vi "z_N[Psi_tau,tau_0,T,W,t_0]_Analytical.vi"(4 "Use z[0]":bool, 5 "tau_0":ext, 6 "t0":ext, 7 "Harmonic f":ext, 8 "N":i32, 9 "W":ext, 10 "T":ext, 11 "tau":ext) -> (3 "z_n,N,W(tau,tau_0)":cxt)   [LabVIEW 2019]
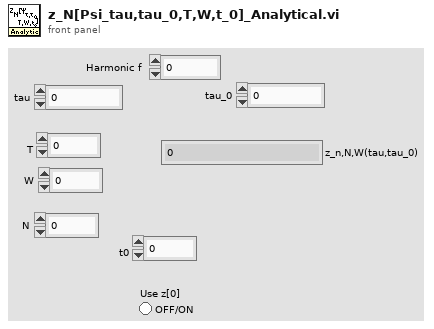
[diagram p1: front panel]
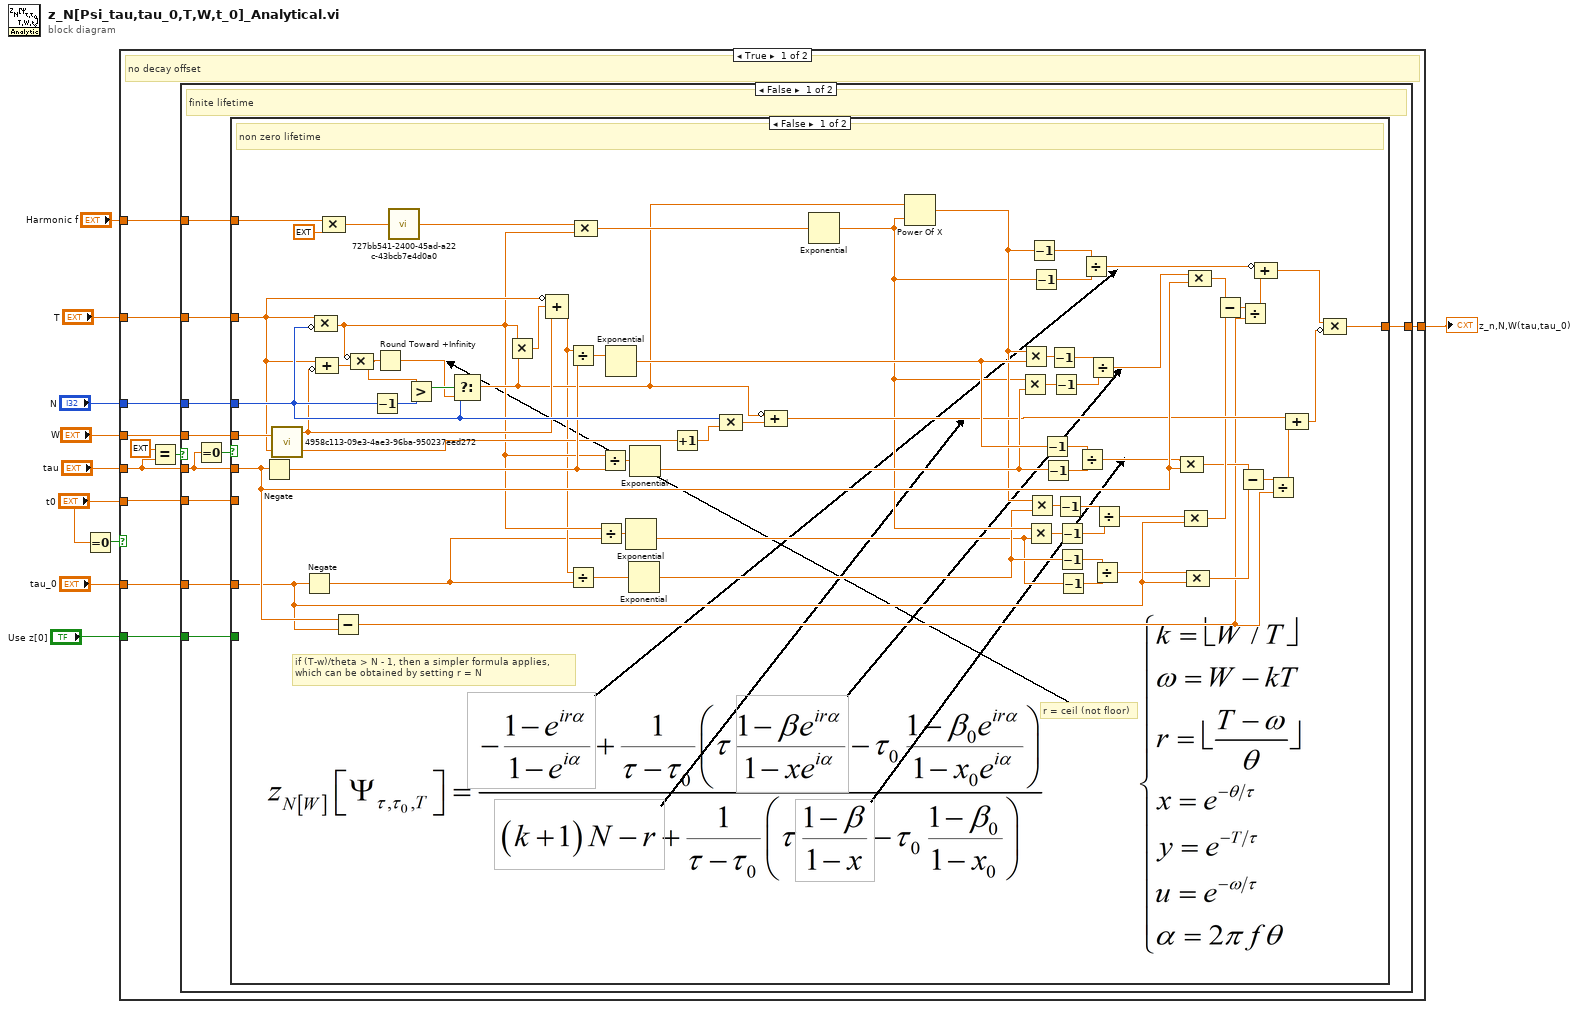
[diagram p0: block diagram]
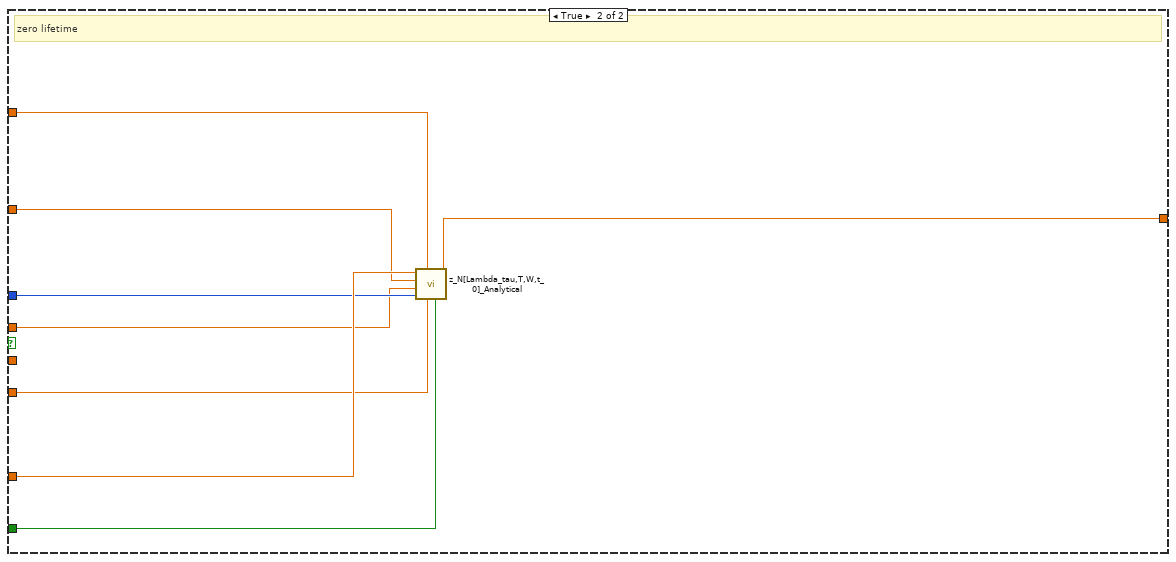
[diagram p2: hidden frame]
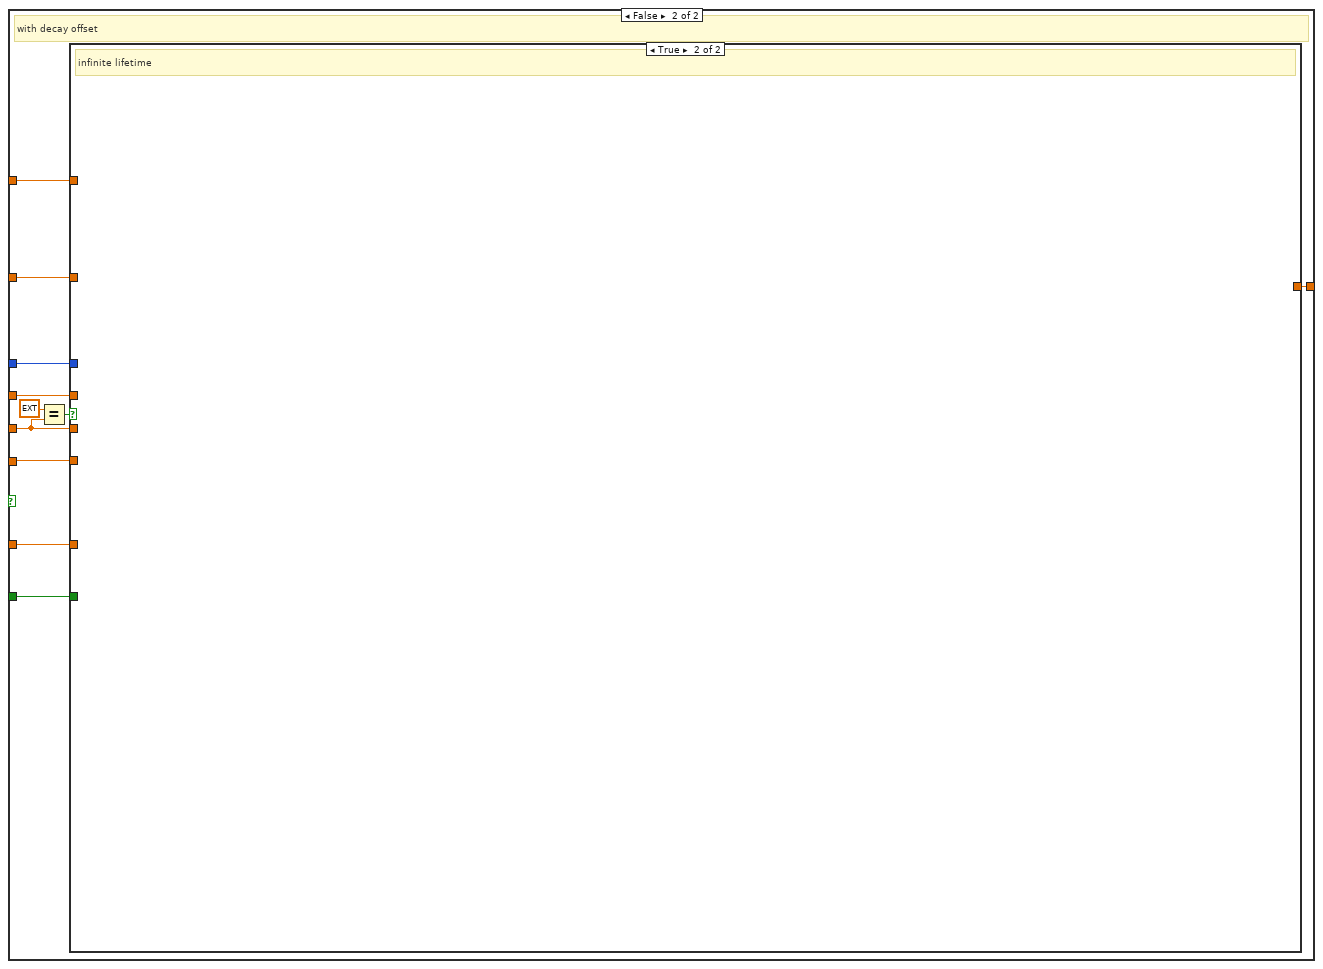
[diagram p4: hidden frame]
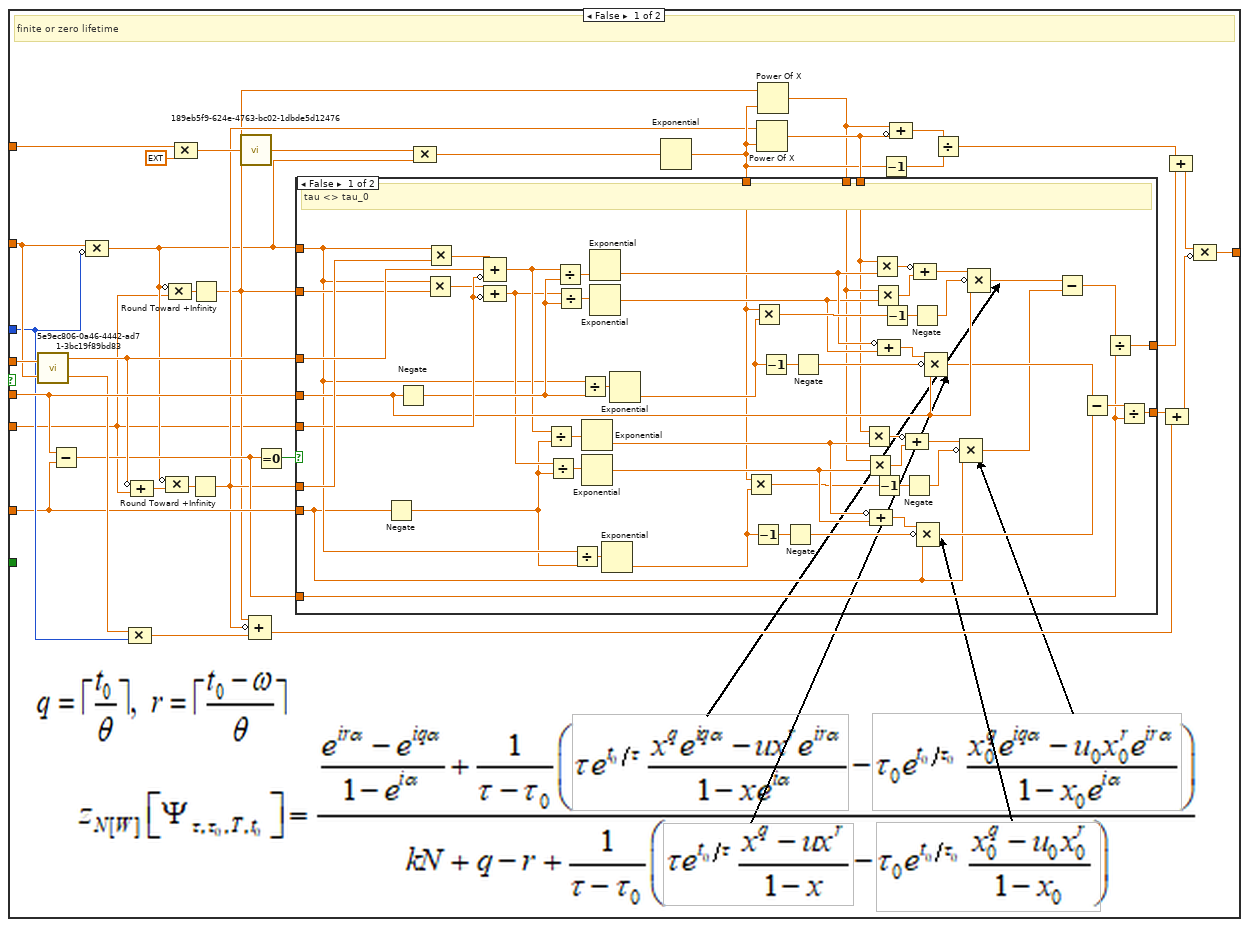
[diagram p5: hidden frame]
diagram:
  n1 = Equal To 0?(x="t0") -> (x = 0?=w3:bool)
  n2 = case shown="True" w3 {
    tunnel: "tau" -> [w16 w112]
    tunnel: "Harmonic f" -> [w21 w117]
    tunnel: [w20 w116] -> w8
    tunnel: "W" -> [w19 w115]
    tunnel: "T" -> [w17 w113]
    tunnel: "N" -> [w18 w114]
    tunnel: "t0" -> [w11 w107]
    tunnel: "Use z[0]" -> [w13 w109]
    tunnel: "tau_0" -> [w12 w108]
    frame True {
      # "no decay offset"
      n3 = Equal?(x=ext inf, y=w16) -> (x = y?=w14:bool)
      n4 = case shown="False" w14 {
        tunnel: w21 -> [w26 _]
        tunnel: [w31 _] -> w20
        tunnel: w19 -> [w30 _]
        tunnel: w18 -> [w29 _]
        tunnel: w17 -> [w28 _]
        tunnel: w16 -> [w27 _]
        tunnel: w13 -> [w24 _]
        tunnel: w12 -> [w23 _]
        tunnel: w11 -> [w22 _]
        frame False {
          # "finite lifetime"
          n5 = Equal To 0?(x=w27) -> (x = 0?=w25:bool)
          n6 = case shown="False" w25 {
            tunnel: [w98 w99] -> w31
            tunnel: w30 -> [w97 w102]
            tunnel: w29 -> [w96 w104]
            tunnel: w28 -> [w95 w103]
            tunnel: w27 -> [w94 _]
            tunnel: w26 -> [w93 w106]
            tunnel: w24 -> [_ w100]
            tunnel: w23 -> [w92 w105]
            tunnel: w22 -> [_ w101]
            frame False {
              # "r = ceil (not floor)"
              # "if (T-w)/theta > N - 1, then a simpler formula applies,\nwhich can be obtained by setting r = N"
              # "non zero lifetime"
              n7 = Negate(x=w94) -> (-x=w78:ext)
              n8 = call "4958c113-09e3-4ae3-96ba-950237eed272.vi"("y"=w95, "x"=w97) -> ("E(x/y)"=w62:ext, "x - E(x/y)y"=w79:ext)
              n9 = Negate(x=w92) -> (-x=w44:ext)
              n10 = Compound Arithmetic op=MULTIPLY(w95, invert w96) -> (w58:ext)
              n11 = Compound Arithmetic op=ADD(w95, invert w79) -> (w80:ext)
              n12 = Compound Arithmetic op=MULTIPLY(w93, ext 6.283185307179586477) -> (w33:ext)
              n13 = Subtract(x=w94, y=w92) -> (x-y=w35:ext)
              n14 = Compound Arithmetic op=MULTIPLY(invert w58, w80) -> (w72:ext)
              n15 = Decrement(x=w96) -> (x-1=w76:i32)
              n16 = Round Toward +Infinity(x=w72) -> (ceil(x): smallest int >= x=w74:ext)
              n17 = call "727bb541-2400-45ad-a22c-43bcb7e4d0a0.vi"("x (1)"=w33) -> ("ix"=w32:cxt)
              n18 = Greater?(x=w72, y=w76) -> (0:w75:bool)
              n19 = Select(t=w96, s=w75, f=w74) -> (s? t:f=w73:ext)
              n20 = Multiply(x=w58, y=w73) -> (x*y=w65:ext)
              n21 = Compound Arithmetic op=ADD(invert w95, w65, w79) -> (w57:ext)
              n22 = Divide(x=w57, y=w78) -> (x/y=w64:ext)
              n23 = Divide(x=w57, y=w44) -> (x/y=w56:ext)
              n24 = Compound Arithmetic op=MULTIPLY(w32, w58) -> (w81:cxt)
              n25 = Divide(x=w58, y=w44) -> (x/y=w59:ext)
              n26 = Divide(x=w58, y=w78) -> (x/y=w63:ext)
              n27 = Exponential(1:w64) -> (0:w89:ext)
              n28 = Exponential(1:w59) -> (0:w40:ext)
              n29 = Exponential(1:w56) -> (0:w41:ext)
              n30 = Exponential(1:w63) -> (0:w86:ext)
              n31 = Increment(x=w62) -> (x+1=w60:ext)
              n32 = Compound Arithmetic op=MULTIPLY(w96, w60) -> (w61:ext)
              n33 = Compound Arithmetic op=ADD(invert w73, w61) -> (w85:ext)
              n34 = Exponential(1:w81) -> (0:w48:cxt)
              n35 = Power Of X(1:w48, 2:w73) -> (0:w49:cxt)
              n36 = Multiply(x=w48, y=w86) -> (x*y=w69:cxt)
              n37 = Multiply(x=w49, y=w89) -> (x*y=w68:cxt)
              n38 = Multiply(x=w48, y=w40) -> (x*y=w53:cxt)
              n39 = Multiply(x=w49, y=w41) -> (x*y=w52:cxt)
              n40 = Decrement(x=w49) -> (x-1=w77:cxt)
              n41 = Decrement(x=w48) -> (x-1=w84:cxt)
              n42 = Decrement(x=w89) -> (x-1=w67:ext)
              n43 = Decrement(x=w86) -> (x-1=w66:ext)
              n44 = Decrement(x=w68) -> (x-1=w71:cxt)
              n45 = Decrement(x=w69) -> (x-1=w70:cxt)
              n46 = Decrement(x=w52) -> (x-1=w55:cxt)
              n47 = Decrement(x=w53) -> (x-1=w54:cxt)
              n48 = Decrement(x=w41) -> (x-1=w50:ext)
              n49 = Decrement(x=w40) -> (x-1=w51:ext)
              n50 = Divide(x=w67, y=w66) -> (x/y=w88:ext)
              n51 = Divide(x=w77, y=w84) -> (x/y=w83:cxt)
              n52 = Divide(x=w71, y=w70) -> (x/y=w91:cxt)
              n53 = Divide(x=w50, y=w51) -> (x/y=w39:ext)
              n54 = Divide(x=w55, y=w54) -> (x/y=w47:cxt)
              n55 = Compound Arithmetic op=MULTIPLY(w88, w94) -> (w38:ext)
              n56 = Compound Arithmetic op=MULTIPLY(w47, w92) -> (w45:cxt)
              n57 = Compound Arithmetic op=MULTIPLY(w39, w92) -> (w37:ext)
              n58 = Compound Arithmetic op=MULTIPLY(w91, w94) -> (w46:cxt)
              n59 = Subtract(x=w46, y=w45) -> (x-y=w43:cxt)
              n60 = Subtract(x=w38, y=w37) -> (x-y=w36:ext)
              n61 = Divide(x=w43, y=w35) -> (x/y=w42:cxt)
              n62 = Compound Arithmetic op=ADD(invert w83, w42) -> (w90:cxt)
              n63 = Divide(x=w36, y=w35) -> (x/y=w34:ext)
              n64 = Compound Arithmetic op=ADD(w85, w34) -> (w82:ext)
              n65 = Compound Arithmetic op=MULTIPLY(w90, invert w82) -> (w98:cxt)
            }
            frame True {
              # "zero lifetime"
              n66 = call "z_N[Lambda_tau,T,W,t_0]_Analytical.vi"("Use z[0]"=w100, "t0"=w101, "Harmonic f"=w106, "N"=w104, "W"=w102, "T"=w103, "tau"=w105) -> ("z_n,N,W(tau)"=w99:cxt)  [unwired: 4 in]
            }
          }
        }
        frame True {
          # "infinite lifetime"
        }
      }
    }
    frame False {
      # "with decay offset"
      n67 = Equal?(x=ext inf, y=w112) -> (x = y?=w110:bool)
      n68 = case shown="True" w110 {
        tunnel: w117 -> [w148 _]
        tunnel: [w151 _] -> w116
        tunnel: w115 -> [w150 _]
        tunnel: w114 -> [w133 _]
        tunnel: w113 -> [w149 _]
        tunnel: w112 -> [w134 _]
        tunnel: w109 -> [_ _]
        tunnel: w108 -> [w130 _]
        tunnel: w107 -> [w118 _]
        frame False {
          # "finite or zero lifetime"
          n69 = call "5e9ec806-0a46-4442-ad71-3bc19f89bd83.vi"("y"=w149, "x"=w150) -> ("E(x/y)"=w132:ext, "x - E(x/y)y"=w129:ext)
          n70 = Subtract(x=w134, y=w130) -> (x-y=w123:ext)
          n71 = Compound Arithmetic op=MULTIPLY(w149, invert w133) -> (w119:ext)
          n72 = Compound Arithmetic op=MULTIPLY(w132, w133) -> (w126:ext)
          n73 = Compound Arithmetic op=ADD(invert w129, w118) -> (w127:ext)
          n74 = Compound Arithmetic op=MULTIPLY(invert w119, w127) -> (w128:ext)
          n75 = Compound Arithmetic op=MULTIPLY(invert w119, w118) -> (w131:ext)
          n76 = Compound Arithmetic op=MULTIPLY(w148, ext 6.283185307179586477) -> (w139:ext)
          n77 = Round Toward +Infinity(x=w128) -> (ceil(x): smallest int >= x=w122:ext)
          n78 = Round Toward +Infinity(x=w131) -> (ceil(x): smallest int >= x=w121:ext)
          n79 = call "189eb5f9-624e-4763-bc02-1dbde5d12476.vi"("x (1)"=w139) -> ("ix"=w138:cxt)
          n80 = Compound Arithmetic op=ADD(w121, invert w122, w126) -> (w124:ext)
          n81 = Equal To 0?(x=w123) -> (x = 0?=w125:bool)
          n82 = Compound Arithmetic op=MULTIPLY(w138, w119) -> (w142:cxt)
          n83 = Exponential(1:w142) -> (0:w136:cxt)
          n84 = Power Of X(1:w136, 2:w122) -> (0:w137:cxt)
          n85 = Power Of X(1:w136, 2:w121) -> (0:w120:cxt)
          n86 = case shown="False" w125 {
            tunnel: [w202 _] -> w141
            tunnel: [w200 _] -> w140
            tunnel: w137 -> [w155 _]
            tunnel: w136 -> [w157 _]
            tunnel: w134 -> [w181 _]
            tunnel: w119 -> [w159 _]
            tunnel: w130 -> [w152 _]
            tunnel: w129 -> [w199 _]
            tunnel: w123 -> [w198 _]
            tunnel: w122 -> [w197 _]
            tunnel: w121 -> [w194 _]
            tunnel: w118 -> [w195 _]
            tunnel: w120 -> [w156 _]
            frame False {
              # "tau <> tau_0"
              n87 = Negate(x=w152) -> (-x=w158:ext)
              n88 = Negate(x=w181) -> (-x=w192:ext)
              n89 = Multiply(x=w159, y=w194) -> (x*y=w193:ext)
              n90 = Multiply(x=w159, y=w197) -> (x*y=w206:ext)
              n91 = Compound Arithmetic op=ADD(w206, w199, invert w195) -> (w161:ext)
              n92 = Compound Arithmetic op=ADD(w193, invert w195) -> (w160:ext)
              n93 = Divide(x=w161, y=w158) -> (x/y=w162:ext)
              n94 = Divide(x=w160, y=w158) -> (x/y=w165:ext)
              n95 = Divide(x=w161, y=w192) -> (x/y=w205:ext)
              n96 = Divide(x=w160, y=w192) -> (x/y=w191:ext)
              n97 = Divide(x=w159, y=w158) -> (x/y=w163:ext)
              n98 = Divide(x=w159, y=w192) -> (x/y=w204:ext)
              n99 = Exponential(1:w162) -> (0:w171:ext)
              n100 = Exponential(1:w165) -> (0:w172:ext)
              n101 = Exponential(1:w205) -> (0:w184:ext)
              n102 = Exponential(1:w191) -> (0:w183:ext)
              n103 = Exponential(1:w163) -> (0:w174:ext)
              n104 = Exponential(1:w204) -> (0:w180:ext)
              n105 = Multiply(x=w157, y=w174) -> (x*y=w168:cxt)
              n106 = Decrement(x=w174) -> (x-1=w175:ext)
              n107 = Multiply(x=w157, y=w180) -> (x*y=w188:cxt)
              n108 = Decrement(x=w180) -> (x-1=w179:ext)
              n109 = Negate(x=w175) -> (-x=w176:ext)
              n110 = Negate(x=w179) -> (-x=w178:ext)
              n111 = Multiply(x=w155, y=w171) -> (x*y=w164:cxt)
              n112 = Multiply(x=w156, y=w172) -> (x*y=w166:cxt)
              n113 = Compound Arithmetic op=ADD(invert w171, w172) -> (w173:ext)
              n114 = Multiply(x=w155, y=w184) -> (x*y=w196:cxt)
              n115 = Multiply(x=w156, y=w183) -> (x*y=w190:cxt)
              n116 = Decrement(x=w168) -> (x-1=w169:cxt)
              n117 = Compound Arithmetic op=ADD(invert w184, w183) -> (w182:ext)
              n118 = Decrement(x=w188) -> (x-1=w187:cxt)
              n119 = Negate(x=w169) -> (-x=w170:cxt)
              n120 = Compound Arithmetic op=ADD(invert w164, w166) -> (w167:cxt)
              n121 = Negate(x=w187) -> (-x=w186:cxt)
              n122 = Compound Arithmetic op=ADD(invert w196, w190) -> (w189:cxt)
              n123 = Compound Arithmetic op=MULTIPLY(w173, invert w176, w152) -> (w153:ext)
              n124 = Compound Arithmetic op=MULTIPLY(w182, invert w178, w181) -> (w177:ext)
              n125 = Compound Arithmetic op=MULTIPLY(w167, invert w170, w152) -> (w154:cxt)
              n126 = Compound Arithmetic op=MULTIPLY(w189, invert w186, w181) -> (w185:cxt)
              n127 = Subtract(x=w185, y=w154) -> (x-y=w203:cxt)
              n128 = Subtract(x=w177, y=w153) -> (x-y=w201:ext)
              n129 = Divide(x=w203, y=w198) -> (x/y=w202:cxt)
              n130 = Divide(x=w201, y=w198) -> (x/y=w200:ext)
            }
            frame True {
              # "tau = tau_0"
            }
          }
          n131 = Decrement(x=w136) -> (x-1=w145:cxt)
          n132 = Compound Arithmetic op=ADD(w120, invert w137) -> (w135:cxt)
          n133 = Divide(x=w135, y=w145) -> (x/y=w144:cxt)
          n134 = Compound Arithmetic op=ADD(w140, w124) -> (w143:ext)
          n135 = Compound Arithmetic op=ADD(w144, w141) -> (w147:cxt)
          n136 = Compound Arithmetic op=MULTIPLY(w147, invert w143) -> (w151:cxt)
        }
        frame True {
          # "infinite lifetime"
        }
      }
    }
  }
  "z_n,N,W(tau,tau_0)" <- w8
